vi "U8 to Bit String.vi"(10 "U8 in":u8[](array[numeric])) -> (2 "String out":string)   [LabVIEW 2019]
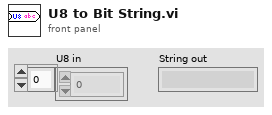
[diagram p1: front panel]
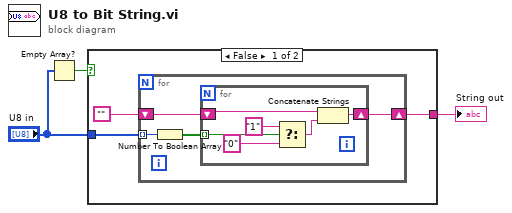
[diagram p0: block diagram]
diagram:
  n1 = Empty Array?(array="U8 in") -> (empty?=w2:bool)
  n2 = case shown="False" w2 {
    tunnel: "U8 in" -> [w6 _]
    tunnel: [w5 _] -> w3
    frame False {
      n3 = for {
        tunnel: w6 -> [w10] mode=indexing
        shift-right: [w8] -> w5
        shift-left: "" -> [w9]
        n4 = Number To Boolean Array(number=w10) -> (Boolean array=w7:bool[])
        n5 = for {
          tunnel: w7 -> [w11] mode=indexing
          shift-right: [w13] -> w8
          shift-left: w9 -> [w12]
          n6 = Select(t="1", s=w11, f="0") -> (s? t:f=w16:string)
          n7 = Concatenate Strings(w12, w16) -> (w13:string)
        }
      }
    }
    frame True {
    }
  }
  "String out" <- w3
